vi "SingleFileCopy Example.vi"() -> ()   [LabVIEW 2013]
uses:
  <vilib>/LabVIEW Open Source Project/Cron Scheduler/Job/Job Report -- cluster.ctl
  Job.SingleFileCopy/FileCopy Job Configuration -- cluster.ctl
  <vilib>/LabVIEW Open Source Project/Cron Scheduler/Job/Job.lvclass/Job.ctl
  <vilib>/LabVIEW Open Source Project/Cron Scheduler/JobReport/JobReport.lvclass/JobReport.ctl
  <vilib>/LabVIEW Open Source Project/Cron Scheduler/Job/Job.lvclass
  <vilib>/LabVIEW Open Source Project/Cron Scheduler/Cron/Create Cron Expression.vi
  <vilib>/LabVIEW Open Source Project/Cron Scheduler/Cron/Compute Next Cron.vi
  <vilib>/LabVIEW Open Source Project/Cron Scheduler/Cron.Quartz/Cron.Quartz.lvclass
  <vilib>/LabVIEW Open Source Project/Cron Scheduler/openCron.lvlib
  <vilib>/LabVIEW Open Source Project/Cron Scheduler/JobReport/JobReport.lvclass
  Job.SingleFileCopy/Job.SingleFileCopy.lvclass
panel:
  out "exception message":string
  in  "FileCopy Job Config":T1={"overwrite?"=TRUE}
  out "% Complete":dbl
  out "last error":errorcluster
  in  "Kill Job":bool
  in  "Abort Job":bool
  out "Job Report":T2
  out "Map":variant
  in  "Cron Expression":string="0/10 * * ? * *"
  out "syntax valid?":bool
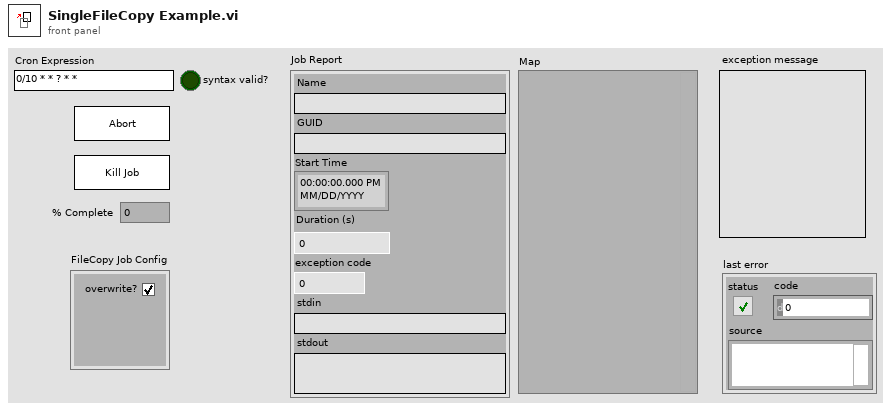
[diagram p1: front panel]
types:
  T1 = typedef "Job.SingleFileCopy.lvclass/FileCopy Job Configuration -- cluster.ctl" = cluster{"overwrite?":bool}
  T2 = typedef "openCronJob.lvlib/JobReport.lvclass/Job Report -- cluster.ctl" = cluster{"Name":string, "GUID":string, "Start Time":timestamp, "Duration (s)":dbl, "exception code":i32, "stdin":string, "stdout":string}
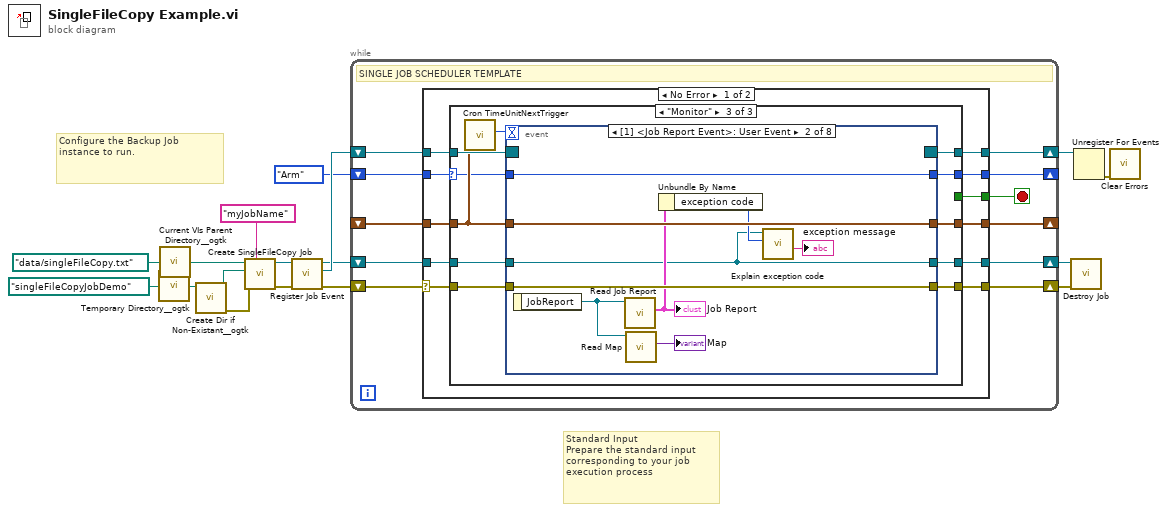
[diagram p0: block diagram]
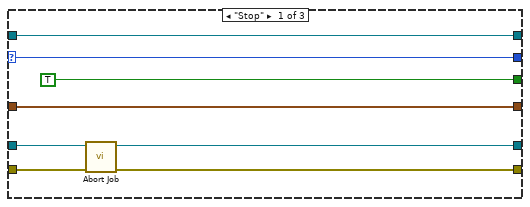
[diagram p2: hidden frame]
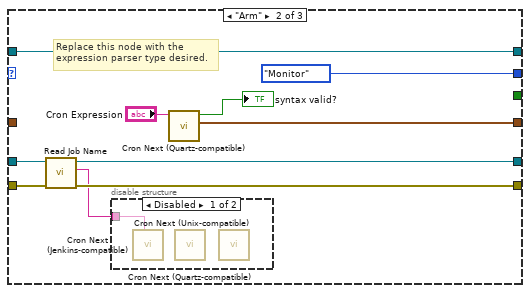
[diagram p3: hidden frame]
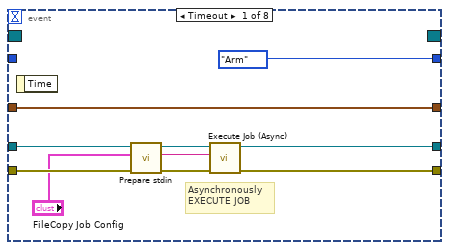
[diagram p5: hidden frame]
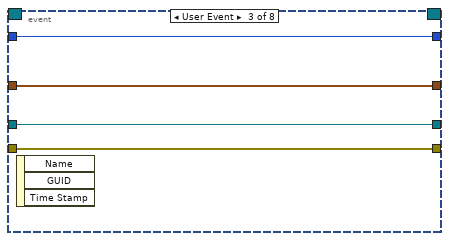
[diagram p6: hidden frame]
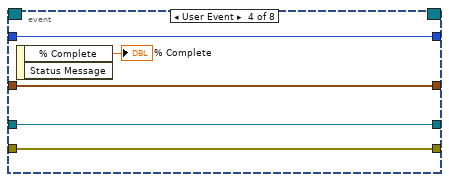
[diagram p7: hidden frame]
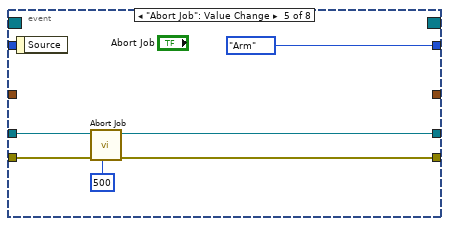
[diagram p8: hidden frame]
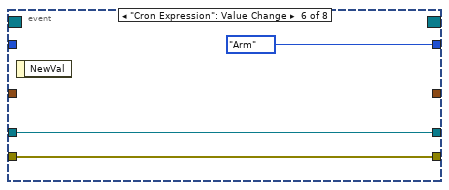
[diagram p9: hidden frame]
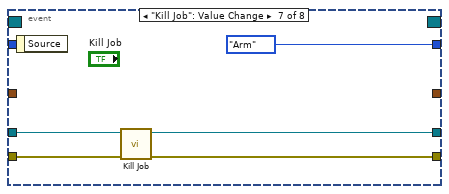
[diagram p10: hidden frame]
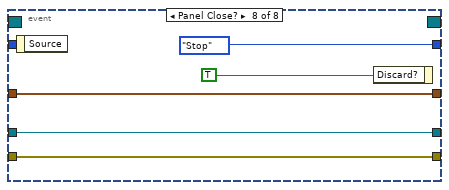
[diagram p11: hidden frame]
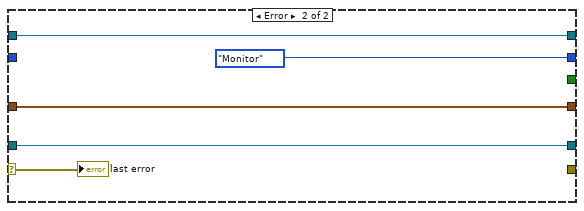
[diagram p12: hidden frame]
diagram:
  # "Standard Input\nPrepare the standard input corresponding to your job execution process"
  # "Configure the Backup Job instance to run."
  n1 = call <userlib>:"Temporary Directory__ogtk.vi"("Relative path (.)"=path "singleFileCopyJobDemo") -> ("Temporary Directory (+ Relative)"=w3:path)
  n2 = call <userlib>:"Current VIs Parent Directory__ogtk.vi"("Relative path (.)"=path "data/singleFileCopy.txt") -> ("Parent Directory (+ Relative)"=w5:path)  [unwired: 4 in]
  n3 = call <userlib>:"Create Dir if Non-Existant__ogtk.vi"("Directory Path"=w3) -> ("error out"=w1:errorcluster, "dup Directory Path"=w2:path)  [unwired: 8 in, 1 out]
  n4 = call "Create SingleFileCopy Job.vi"("Job Name"="myJobName", "error in (no error)"=w1, "Destination"=w2, "Source"=w5) -> ("error out"=w8:errorcluster, "Job.SingleFileCopy"=w9:refnum<class "Job.SingleFileCopy.lvclass">)  [unwired: 6 in]
  n5 = call <vilib>:"Register Job Event.vi"("Job in"=w9) -> ("Job Event Registration"=w16:refnum<event-registration>, "Job out"=w14:refnum<class "Job.SingleFileCopy.lvclass">)  [unwired: 9 in]
  n6 = while {
    shift-right: [w26] -> _
    shift-left: _ -> [w27]
    shift-right: [w24] -> _
    shift-left: enum16{"Arm", "Stop", "Monitor"}."Arm" -> [w25]
    shift-right: [w21] -> w11
    shift-left: w16 -> [w22]
    shift-right: [w19] -> w13
    shift-left: w14 -> [w20]
    shift-right: [w18] -> w15
    shift-left: w8 -> [w17]
    stop <- w23 stop-if-true
    # "SINGLE JOB SCHEDULER TEMPLATE"
    n7 = case shown="No Error" w17 {
      selector: w17 -> [w28 w116]
      tunnel: w27 -> [w38 w118]
      tunnel: [w37 w118] -> w26
      tunnel: w25 -> [w36 _]
      tunnel: [w35 enum16{"Arm", "Stop", "Monitor"}."Monitor"] -> w24
      tunnel: [w34 _] -> w23
      tunnel: w22 -> [w33 w120]
      tunnel: [w32 w120] -> w21
      tunnel: w20 -> [w31 w117]
      tunnel: [w30 w117] -> w19
      tunnel: [w29 _] -> w18
      frame No Error {
        n8 = case shown="\"Monitor\"" w36 {
          selector: w36 -> [w46 _ w60]
          tunnel: w38 -> [w44 _ w63]
          tunnel: [w44 w55 w65] -> w37
          tunnel: [w46 enum16{"Arm", "Stop", "Monitor"}."Monitor" w66] -> w35
          tunnel: [TRUE _ _] -> w34
          tunnel: w33 -> [w43 w56 w68]
          tunnel: [w43 w56 w67] -> w32
          tunnel: w31 -> [w42 w49 w62]
          tunnel: [w41 w48 w61] -> w30
          tunnel: w28 -> [w40 w51 w59]
          tunnel: [w39 w50 w58] -> w29
          frame "Stop" {
            n9 = call <vilib>:"Abort Job.vi"("error in (no error)"=w40, "Job in"=w42) -> ("error out"=w39:errorcluster, "Job out"=w41:refnum<class "Job.SingleFileCopy.lvclass">)  [unwired: 5 in, 3 out]
          }
          frame "Arm" {
            # "Replace this node with the\nexpression parser type desired."
            n10 = call <vilib>:"Read Job Name.vi"("error in (no error)"=w51, "Job in"=w49) -> ("error out"=w50:errorcluster, "Name"=w47:string, "Job out"=w48:refnum<class "Job.SingleFileCopy.lvclass">)  [unwired: 7 in]
            n11 = disable-structure shown="Disabled" {
              disable-tunnel: w47 -> [w57 _]
              frame Disabled {
                n12 = call <vilib>:"Cron Next (Jenkins-compatible).vi"("Job Name"=w57) -> ()  [unwired: 8 in, 3 out]
                n13 = call <vilib>:"Cron Next (Quartz-compatible).vi"() -> ()  [unwired: 9 in, 3 out]
                n14 = call <vilib>:"Cron Next (Unix-compatible).vi"() -> ()  [unwired: 9 in, 3 out]
              }
              frame Enabled {
              }
            }
            n15 = call <vilib>:"Cron Next (Quartz-compatible).vi"("Cron Expression"="Cron Expression") -> ("Next Occurence"=w55:timestamp, "syntax valid?"=→"syntax valid?":bool)  [unwired: 8 in, 1 out]
          }
          frame "Monitor" {
            n16 = call <vilib>:"Cron TimeUnitNextTrigger.vi"("Next Occurence"=w63) -> ("next event (ms)"=w64:i32)  [unwired: 10 in]
            n17 = event shown="[1] <Job Report Event>: User Event" {
              selector: w68 -> [_ _ _ _ _ _ _ _]
              dyn-events: [_ _ _ _ _ _ _ _] -> w67
              timeout: w64 -> [_ _ _ _ _ _ _ _]
              tunnel: [enum16{"Arm", "Stop", "Monitor"}."Arm" w86 w90 w95 enum16{"Arm", "Stop", "Monitor"}."Arm" enum16{"Arm", "Stop", "Monitor"}."Arm" enum16{"Arm", "Stop", "Monitor"}."Arm" enum16{"Arm", "Stop", "Monitor"}."Stop"] -> w66
              tunnel: [w75 w87 w91 w96 _ _ _ w113] -> w65
              tunnel: w63 -> [w75 w87 w91 w96 _ _ _ w113]
              tunnel: w62 -> [w74 w79 w89 w94 w101 w104 w109 w112]
              tunnel: [w77 w79 w89 w94 w100 w104 w108 w112] -> w61
              tunnel: w60 -> [_ w86 w90 w95 _ _ _ _]
              tunnel: w59 -> [w72 w85 w88 w93 w98 w103 w107 w111]
              tunnel: [w76 w85 w88 w93 w97 w103 w106 w111] -> w58
              event Timeout {
                # "Asynchronously\nEXECUTE JOB"
                n18 = event-data() -> ()  [unwired: 1 in, 1 out]
                n19 = call "Prepare stdin.vi"("error in (no error)"=w72, "FileCopy Job Config"="FileCopy Job Config", "Job.SingleFileCopy in"=w74) -> ("error out"=w71:errorcluster, "Stdin"=w69:string, "Job.SingleFileCopy out"=w73:refnum<class "Job.SingleFileCopy.lvclass">)  [unwired: 6 in]
                n20 = call <vilib>:"Execute Job (Async).vi"("error in (no error)"=w71, "stdin"=w69, "Job in"=w73) -> ("error out"=w76:errorcluster, "Job out"=w77:refnum<class "Job.SingleFileCopy.lvclass">)  [unwired: 6 in, 1 out]
              }
              event User Event {
                n21 = event-data() -> ("JobReport"=w84:refnum<class "JobReport.lvclass">)  [unwired: 1 in]
                n22 = call <vilib>:"Read Job Report.vi"("JobReport in"=w84) -> ("Job Report"=w82:T2)  [unwired: 8 in, 2 out]
                "Job Report" <- w82
                n23 = call <vilib>:"Read Map.vi"("JobReport in"=w84) -> ("Map"=→"Map":variant)  [unwired: 8 in, 2 out]
                n24 = Unbundle By Name(w82) -> ("exception code"=w80:i32)
                n25 = call <vilib>:"Explain exception code.vi"("exception"=w80, "Job type"=w79) -> ("exception message"=→"exception message":string)  [unwired: 7 in, 2 out]
              }
              event User Event {
                n26 = event-data() -> ()  [unwired: 1 in, 3 out]
              }
              event User Event {
                n27 = event-data() -> ("% Complete"=→"% Complete":dbl)  [unwired: 1 in, 1 out]
              }
              event "Abort Job": Value Change {
                n28 = event-data() -> ()  [unwired: 1 in, 1 out]
                n29 = call <vilib>:"Abort Job.vi"("timeout (500 ms)"=500, "error in (no error)"=w98, "Job in"=w101) -> ("error out"=w97:errorcluster, "Job out"=w100:refnum<class "Job.SingleFileCopy.lvclass">)  [unwired: 4 in, 3 out]
              }
              event "Cron Expression": Value Change {
                n30 = event-data() -> ()  [unwired: 1 in, 1 out]
              }
              event "Kill Job": Value Change {
                n31 = event-data() -> ()  [unwired: 1 in, 1 out]
                n32 = call <vilib>:"Kill Job.vi"("error in (no error)"=w107, "Job in"=w109) -> ("error out"=w106:errorcluster, "Job out"=w108:refnum<class "Job.SingleFileCopy.lvclass">)  [unwired: 8 in]
              }
              event Panel Close? {
                n33 = event-data() -> ()  [unwired: 1 in, 1 out]
                n34 = event-data("Discard?"=TRUE) -> ()  [unwired: 1 in, 1 out]
              }
            }
          }
        }
      }
      frame Error {
        "last error" <- w116
      }
    }
  }
  n35 = call <vilib>:"Destroy Job.vi"("error in (no error)"=w15, "Job in"=w13) -> ()  [unwired: 8 in, 2 out]
  n36 = Unregister For Events(event registration refnum=w11) -> (error out=w12:errorcluster)  [unwired: 1 in]
  n37 = call <vilib>:"Clear Errors.vi"("error in (no error)"=w12) -> ()  [unwired: 6 in, 1 out]
